vi "Check if Fault or Limit.vi"(8 "error in (no error)":errorcluster, 10 "Ignore Limit Switches?":bool, 11 "Status In":u16 format="%x") -> (0 "error out":errorcluster, 3 "Fault or Limit":bool)   [LabVIEW 2015, in "Tool Module.lvlib"]
uses:
  Tool Module.lvlib
  _Status Bits Typedef.ctl
  Tool Config/Tool Cfg.lvlib
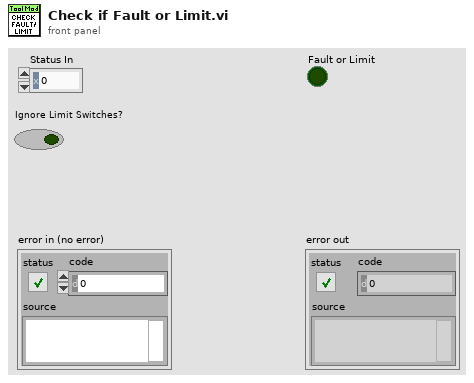
[diagram p1: front panel]
types:
  T1 = typedef "Tool Module.lvlib/_Status Bits Typedef.ctl" = u16
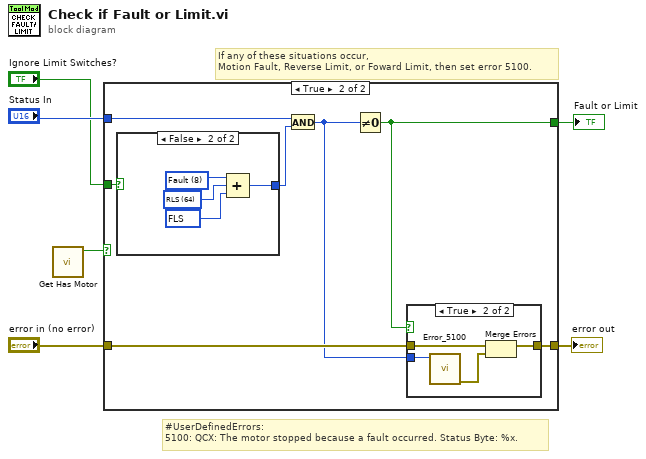
[diagram p0: block diagram]
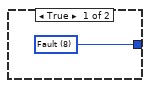
[diagram p3: hidden frame]
diagram:
  # "#UserDefinedErrors:\n5100: QCX: The motor stopped because a fault occurred. Status Byte: %x."
  # "If any of these situations occur, \nMotion Fault, Reverse Limit, or Foward Limit, then set error 5100."
  n1 = call "Get Has Motor.vi"() -> ("Has Motor"=w1:bool)  [unwired: 11 in]
  n2 = case shown="True" w1 {
    tunnel: "error in (no error)" -> [w7 w13]
    tunnel: [w7 w12] -> w3
    tunnel: "Ignore Limit Switches?" -> [_ w11]
    tunnel: "Status In" -> [_ w10]
    tunnel: [_ w9] -> w6
    frame False {
    }
    frame True {
      n3 = case shown="False" w11 {
        tunnel: [w15 w19] -> w14
        frame True {
          w15 = T1 8 items=["PROX1"=1, "PartPresent"=2, "Motion"=4, "Fault"=8, "Switch"=16, "Home"=32, "RLS"=64, "FLS"=128, "PROX2"=256, "INSPECT"=512, "Abort"=1024, "Stop on Limit"=2048] ("_Status bit values--typedef")
        }
        frame False {
          w16 = T1 128 items=["PROX1"=1, "PartPresent"=2, "Motion"=4, "Fault"=8, "Switch"=16, "Home"=32, "RLS"=64, "FLS"=128, "PROX2"=256, "INSPECT"=512, "Abort"=1024, "Stop on Limit"=2048] ("_Status bit values--typedef")
          w17 = T1 64 items=["PROX1"=1, "PartPresent"=2, "Motion"=4, "Fault"=8, "Switch"=16, "Home"=32, "RLS"=64, "FLS"=128, "PROX2"=256, "INSPECT"=512, "Abort"=1024, "Stop on Limit"=2048] ("_Status bit values--typedef")
          w18 = T1 8 items=["PROX1"=1, "PartPresent"=2, "Motion"=4, "Fault"=8, "Switch"=16, "Home"=32, "RLS"=64, "FLS"=128, "PROX2"=256, "INSPECT"=512, "Abort"=1024, "Stop on Limit"=2048] ("_Status bit values--typedef")
          n4 = Compound Arithmetic op=unknown(w18, w17, w16) -> (w19:T1)
        }
      }
      n5 = And(x=w10, y=w14) -> (x .and. y?=w8:T1)
      n6 = Not Equal To 0?(x=w8) -> (x != 0?=w9:bool)
      n7 = case shown="True" w9 {
        tunnel: w13 -> [w20 w24]
        tunnel: [w20 w23] -> w12
        tunnel: w8 -> [_ w21]
        frame False {
        }
        frame True {
          n8 = call "Error_5100.vi"("Status Byte"=w21) -> ("error out"=w22:errorcluster)  [unwired: 10 in]
          n9 = Merge Errors(w24, w22) -> (w23:errorcluster)
        }
      }
    }
  }
  "error out" <- w3
  "Fault or Limit" <- w6
